vi "Read UID.vi"(11 "Base Setup in":refnum<class "Base Setup.lvclass">) -> (2 "UID":string)   [LabVIEW 2025, in "jettl.lvlib" / "Setup.lvlib" / "Base Setup.lvclass"]
uses:
  Base Setup.lvclass
  Base Setup.lvclass/Base Setup.ctl
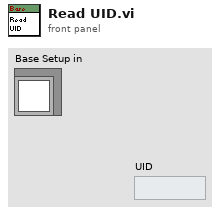
[diagram p1: front panel]
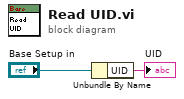
[diagram p0: block diagram]
diagram:
  n1 = Unbundle By Name("Base Setup in") -> ("UID"=→"UID":string)
